vi "Programa de labview DAQ.vi"() -> ()   [LabVIEW 2014]
uses:
  <vilib>/Instr/_visa.llb/Select Event Type.ctl
panel:
  out "Numeric":i32
  in  "milliseconds to wait":u32
  in  "Slide":i32(slide) scale=0.0..100.0
  out "Waveform Chart":u8(graph)
  out "array":string[](array[string])
  out "unsigned 32bit integer":u32[](array[numeric])
  in  "PWM 1":u8(slide)=30 scale=0.0..255.0
  in  "PWM 2":u8(slide)=41 scale=0.0..255.0
  out "ENTRADAS PUERTO D":bool[](array[boolean])
  out "Thermometer":dbl(slide) scale=0.0..255.0
  in  "SALIDAS PUERTO B":bool[](array[boolean])
  out "CONT":dbl
  out "AN6":dbl
  out "AN5":dbl
  out "AN4":dbl
  out "AN3":dbl
  out "AN2":dbl
  out "AN1":dbl
  out "Byte recibido":u16
  out "Byte enviado":u32
  out "Datos recibidos":u8[](array[numeric])
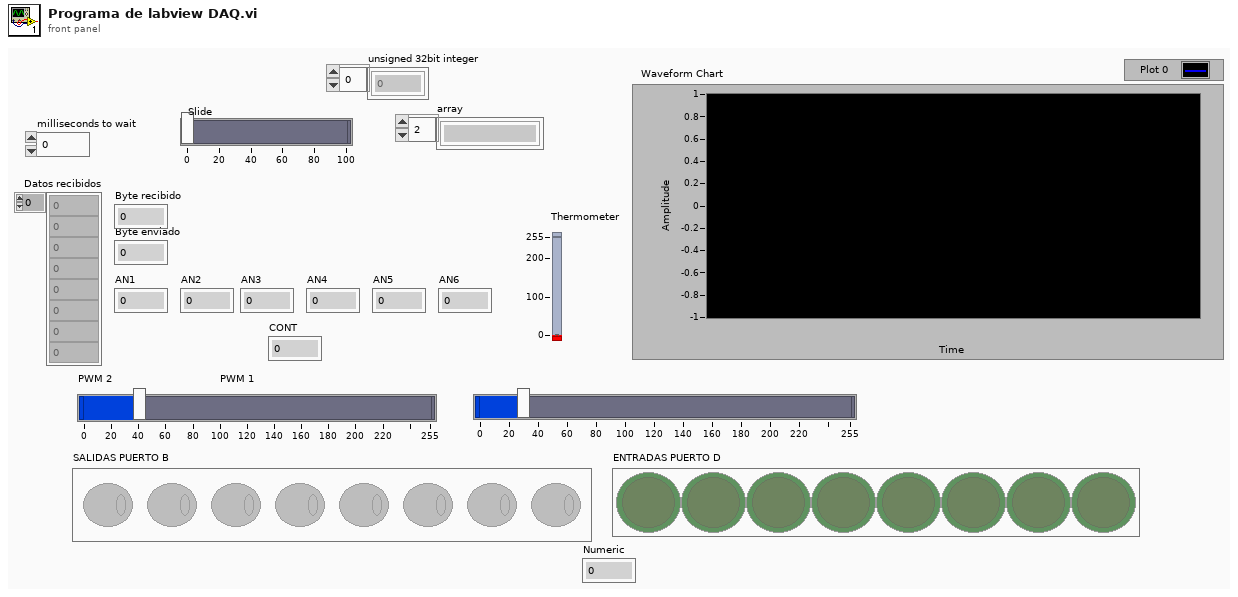
[diagram p1: front panel]
types:
  T1 = typedef "Select Event Type.ctl" = u32
  T2 = cluster{"string":string, "string":string, "string":string}
  T3 = cluster{"data buffer[0]":u8, "data buffer[1]":u8, "data buffer[2]":u8, "data buffer[3]":u8, "data buffer[4]":u8, "data buffer[5]":u8, "data buffer[6]":u8, "data buffer[7]":u8, "data buffer[8]":u8}
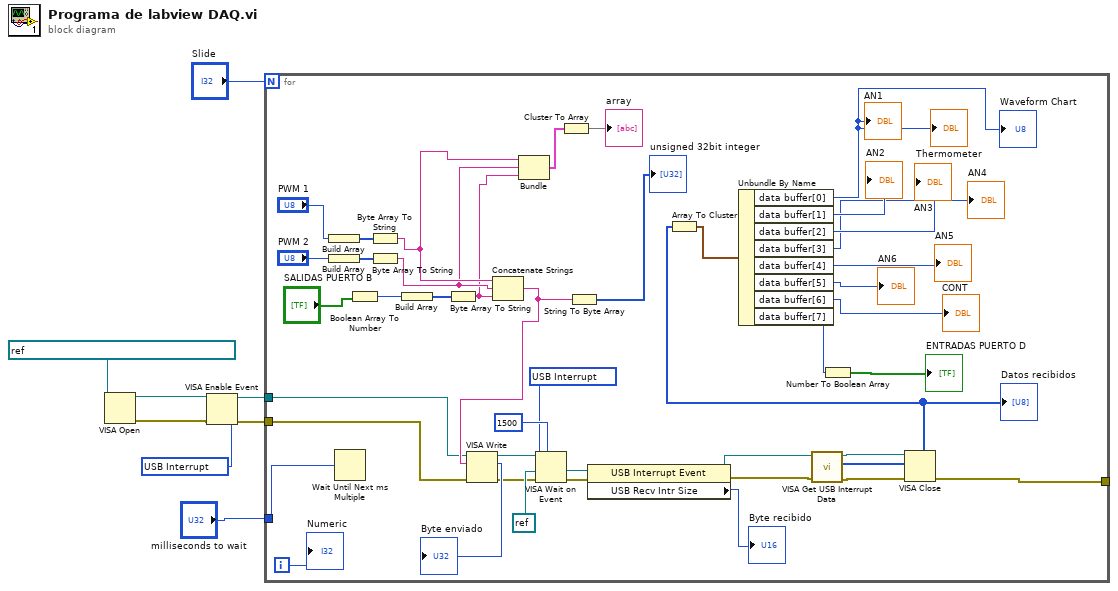
[diagram p0: block diagram]
diagram:
  w7 = T1 1073684535 items=["Service Request"=1073684491, "Trigger"=3221168138, "Clear"=1073684493, "VXI Signal"=1073684512, "VXI/VME Interrupt"=3221168161, "VXI/VME Sysfail"=1073684509, "VXI/VME Sysreset"=1073684510, "GPIB CIC"=1073684498, "GPIB Talk"=1073684499, "GPIB Listen"=1073684500, "PXI Interrupt"=1073684514, "Serial Break"=1073684515, "Serial TermChar"=1073684516, "Serial CTS"=1073684521, "Serial DSR"=1073684522, "Serial DCD"=1073684524, "Serial RI"=1073684526, "Serial Character"=1073684533, "USB Interrupt"=1073684535, "All Enabled"=1073709055] ("Event Type")
  n1 = VISA Open(VISA resource name=refnum<visa-resource-name> "USB0::0x0461::0x0020::NI-VISA-0::RAW") -> (VISA resource name=w6:refnum<visa-resource-name>, error out=w5:errorcluster)  [unwired: 4 in]
  n2 = VISA Enable Event(8:w5, 10:w7, 11:w6) -> (0:w3:errorcluster, 3:w4:refnum<visa-resource-name>)  [unwired: 1 in]
  n3 = for {
    N: "Slide" -> [_]
    tunnel: [w42] -> _
    tunnel: w4 -> [w11]
    tunnel: w3 -> [w10]
    tunnel: "milliseconds to wait" -> [w9]
    i -> [w16]
    w14 = T1 1073684535 items=["Service Request"=1073684491, "Trigger"=3221168138, "Clear"=1073684493, "VXI Signal"=1073684512, "VXI/VME Interrupt"=3221168161, "VXI/VME Sysfail"=1073684509, "VXI/VME Sysreset"=1073684510, "GPIB CIC"=1073684498, "GPIB Talk"=1073684499, "GPIB Listen"=1073684500, "PXI Interrupt"=1073684514, "Serial Break"=1073684515, "Serial TermChar"=1073684516, "Serial CTS"=1073684521, "Serial DSR"=1073684522, "Serial DCD"=1073684524, "Serial RI"=1073684526, "Serial Character"=1073684533, "USB Interrupt"=1073684535, "All Enabled"=1073709055] ("Event Type")
    n4 = Build Array("PWM 1") -> (w28:u8[])
    n5 = Build Array("PWM 2") -> (w26:u8[])
    n6 = Wait Until Next ms Multiple(millisecond multiple=w9) -> ()  [unwired: 1 out]
    n7 = Boolean Array To Number(Boolean array="SALIDAS PUERTO B") -> (number=w44:u32)
    n8 = Byte Array To String(unsigned byte array=w28) -> (string=w24:string)
    n9 = Byte Array To String(unsigned byte array=w26) -> (string=w23:string)
    n10 = Build Array(w44) -> (w45:u32[])
    n11 = Byte Array To String(unsigned byte array=w45) -> (string=w22:string)
    n12 = Concatenate Strings(w24, w23, w22) -> (w19:string)
    n13 = VISA Write(VISA resource name=w11, write buffer=w19, error in (no error)=w10) -> (VISA resource name out=w51:refnum<visa-resource-name>, return count=→"Byte enviado":u32, error out=w13:errorcluster)
    n14 = Bundle("string"=w24, "string"=w23, "string"=w22) -> (w20:T2)  [unwired: 1 in]
    n15 = VISA Wait on Event(7:u32 1500 ("General Settings:Timeout Value"), 8:w13, 9:refnum<visa-resource-name> refnum ("event class (Generic Event)"), 10:w14, 11:w51) -> (0:w50:errorcluster, 1:w41:refnum<visa-resource-name>)  [unwired: 2 out]
    n16 = Cluster To Array(cluster=w20) -> (array=→"array":string[])
    n17 = String To Byte Array(string=w19) -> (unsigned byte array=→"unsigned 32bit integer":u8[])
    n18 = property class="USB Interrupt Event"(reference=w41, error in=w50) -> (reference out=w46:refnum<visa-resource-name>, error out=w47:errorcluster, "USB Recv Intr Size"=→"Byte recibido":u16)
    n19 = call <vilib>:"VISA Get USB Interrupt Data.vi"("error in (no error)"=w47, "VISA USB Intr Event"=w46) -> ("error out"=w43:errorcluster, "data buffer"=w12:u8[], "VISA USB Intr Event out"=w25:refnum<visa-resource-name>)  [unwired: 7 in]
    "Datos recibidos" <- w12
    n20 = Array To Cluster(array=w12) -> (cluster=w39:T3)
    n21 = Unbundle By Name(w39) -> ("data buffer[0]"=→"AN1" →"Thermometer" →"Waveform Chart":u8, "data buffer[1]"=→"AN2":u8, "data buffer[2]"=→"AN3":u8, "data buffer[3]"=→"AN4":u8, "data buffer[4]"=→"AN5":u8, "data buffer[5]"=→"AN6":u8, "data buffer[6]"=→"CONT":u8, "data buffer[7]"=w30:u8)
    n22 = Number To Boolean Array(number=w30) -> (Boolean array=→"ENTRADAS PUERTO D":bool[])
    n23 = VISA Close(VISA resource name=w25, error in (no error)=w43) -> (error out=w42:errorcluster)
    "Numeric" <- w16
  }
